vi "Polynomial Real Zero Counter.vi"(2 "Polynomial":dbl[](array[numeric]) format="%.2f", 3 "end":dbl=1.0 format="%.2f", 4 "start":dbl format="%.2f") -> (0 "error":i32, 1 "number of zeroes":i32)   [LabVIEW 2017, in "NI_Gmath.lvlib"]
doc: "Calculates the number of zeros of a given real polynomial in a real interval without determining of the values of these zeros."
uses:
  <vilib>/gmath/NI_Gmath.lvlib
  <vilib>/Analysis/NI_AALPro.lvlib
  <vilib>/Analysis/NI_AALBase.lvlib
panel:
  # "Example:\n\n start: 0.0\n end: 3.0\n Polynomial: (1.0,-3.0,2.0)"
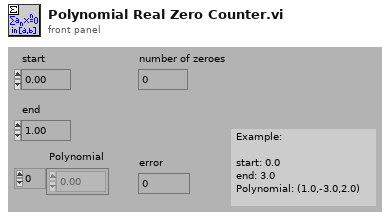
[diagram p1: front panel]
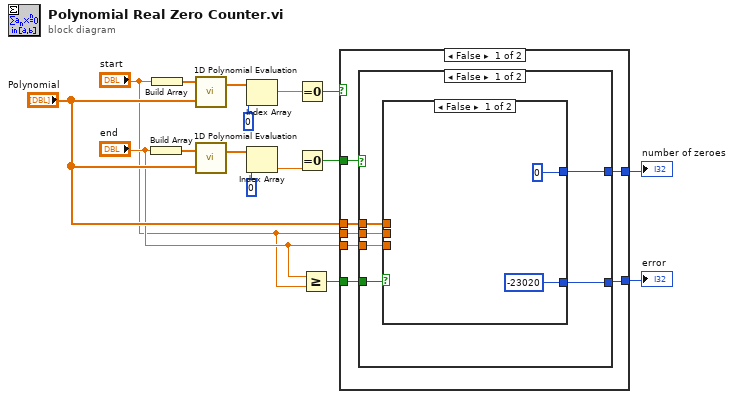
[diagram p0: block diagram]
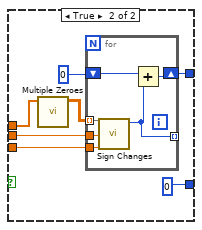
[diagram p2: hidden frame]
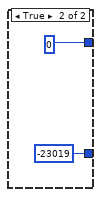
[diagram p3: hidden frame]
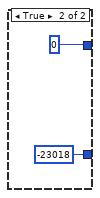
[diagram p4: hidden frame]
diagram:
  n1 = Build Array("end") -> (w16:dbl[])
  n2 = Build Array("start") -> (w15:dbl[])
  n3 = call <vilib>:"1D Polynomial Evaluation.vi"("Coefficients: a"="Polynomial", "X"=w15) -> ("Y"=w14:dbl[])  [unwired: 1 out]
  n4 = call <vilib>:"1D Polynomial Evaluation.vi"("Coefficients: a"="Polynomial", "X"=w16) -> ("Y"=w8:dbl[])  [unwired: 1 out]
  n5 = Index Array(array=w14, index=0) -> (element=w12:dbl)
  n6 = Index Array(array=w8, index=0) -> (element=w7:dbl)
  n7 = Equal To 0?(x=w12) -> (x = 0?=w11:bool)
  n8 = Equal To 0?(x=w7) -> (x = 0?=w6:bool)
  n9 = Greater Or Equal?(x="end", y="start") -> (x >= y?=w1:bool)
  n10 = case shown="False" w11 {
    tunnel: [w22 -23018] -> w10
    tunnel: w6 -> [w23 _]
    tunnel: "Polynomial" -> [w21 _]
    tunnel: "start" -> [w20 _]
    tunnel: "end" -> [w19 _]
    tunnel: [w18 0] -> w4
    tunnel: w1 -> [w17 _]
    frame False {
      n11 = case shown="False" w23 {
        tunnel: [w24 -23019] -> w22
        tunnel: w21 -> [w29 _]
        tunnel: w20 -> [w28 _]
        tunnel: w19 -> [w27 _]
        tunnel: [w26 0] -> w18
        tunnel: w17 -> [w25 _]
        frame False {
          n12 = case shown="False" w25 {
            tunnel: [0 w38] -> w26
            tunnel: w27 -> [_ w37]
            tunnel: w28 -> [_ w36]
            tunnel: w29 -> [_ w33]
            tunnel: [-23020 0] -> w24
            frame False {
            }
            frame True {
              n13 = call <vilib>:"Multiple Zeroes.vi"("p"=w33) -> ("sequence of polynomials"=w35:dbl[][])  [unwired: 10 in]
              n14 = for {
                shift-right: [w40] -> w38
                shift-left: 0 -> [w41]
                tunnel: w35 -> [w44] mode=indexing
                tunnel: w36 -> [w43]
                tunnel: w37 -> [w42]
                tunnel: [w39] -> _ mode=indexing
                n15 = call <vilib>:"Sign Changes.vi"("x1"=w42, "x0"=w43, "f"=w44) -> ("number of roots"=w39:i32)  [unwired: 8 in]
                n16 = Add(x=w41, y=w39) -> (x+y=w40:i32)
              }
            }
          }
        }
        frame True {
        }
      }
    }
    frame True {
    }
  }
  "number of zeroes" <- w4
  "error" <- w10
